vi "Sub P.vi"(9 "VISA resource name":refnum<visa-resource-name>="COM3") -> (1 "实测温度":string="020300010001D5F9")   [LabVIEW 2021]
uses:
  <vilib>/Instr/_visa.llb/VISA Configure Serial Port (Instr).vi
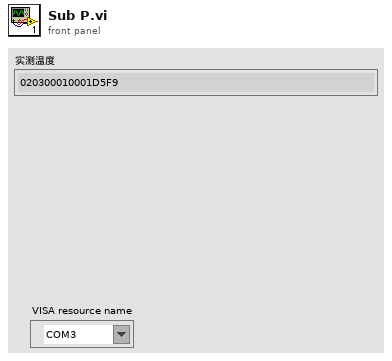
[diagram p1: front panel]
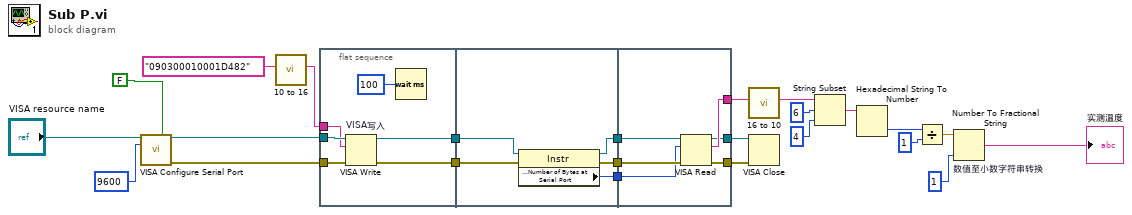
[diagram p0: block diagram]
diagram:
  n1 = call-poly "VISA Configure Serial Port"("VISA resource name"="VISA resource name", "Enable Termination\nChar (T)"=FALSE ("确定按钮"), "baud rate (9600)"=u32 9600) -> ("VISA resource name out"=w17:refnum<visa-resource-name>, "error out"=w16:errorcluster)  [unwired: 11 in]
  n2 = call "10 to 16.vi"("字符串"="090300010001D482" ("写入缓冲区")) -> ("字符串 2"=w15:string)  [unwired: 10 in]
  n3 = flat-sequence {
    tunnel: w17 -> [w30]
    tunnel: w16 -> [w29]
    tunnel: w15 -> [w28]
    tunnel: [w27] -> w14
    tunnel: [w26] -> w13
    tunnel: [w35] -> w20
    tunnel: [w34] -> w19
    tunnel: [w33] -> w18
    tunnel: w14 -> [w32]
    tunnel: w13 -> [w31]
    tunnel: [w41] -> w21
    tunnel: [w40] -> w3
    tunnel: w20 -> [w39]
    tunnel: w19 -> [w38]
    tunnel: w18 -> [w37]
    tunnel: [w36] -> w2
    frame #0 {
      n4 = VISA Write "VISA写入"(VISA resource name=w30, write buffer=w28, error in (no error)=w29) -> (VISA resource name out=w27:refnum<visa-resource-name>, error out=w26:errorcluster)  [unwired: 1 out]
      n5 = Wait (ms)(milliseconds to wait=u32 100 ("baud rate (9600)")) -> ()  [unwired: 1 out]
    }
    frame #1 {
      n6 = property class="Instr"(reference=w32, error in=w31) -> (reference out=w35:refnum<visa-resource-name>, error out=w34:errorcluster, "Serial Settings:Number of Bytes at Serial Port"=w33:u32)
    }
    frame #2 {
      n7 = VISA Read ("VISA读取")(VISA resource name=w39, byte count=w37, error in (no error)=w38) -> (VISA resource name out=w40:refnum<visa-resource-name>, read buffer=w41:string, error out=w36:errorcluster)  [unwired: 1 out]
    }
  }
  n8 = call "16 to 10.vi"("字符串"=w21) -> ("字符串 2"=w12:string)  [unwired: 10 in]
  n9 = VISA Close(VISA resource name=w3, error in (no error)=w2) -> ()  [unwired: 1 out]
  n10 = String Subset(string=w12, offset (0)=u32 6 ("baud rate (9600)"), length (rest)=u32 4 ("baud rate (9600)")) -> (substring=w9:string)
  n11 = Hexadecimal String To Number ("十六进制数字符串至数值转换")(string=w9) -> (number=w8:u32)  [unwired: 2 in, 1 out]
  n12 = Divide(x=w8, y=u32 1 ("baud rate (9600)")) -> (x/y=w6:dbl)
  n13 = Number To Fractional String "数值至小数字符串转换"(number=w6, precision (6)=u32 1 ("baud rate (9600)")) -> (F-format string=→"实测温度":string)  [unwired: 2 in]
